vi "motor.vi"() -> ()   [LabVIEW 2018]
panel:
  out "返回值":string
  out "连接串口":string
  out "移动位置":string
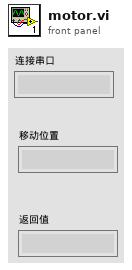
[diagram p1: front panel]
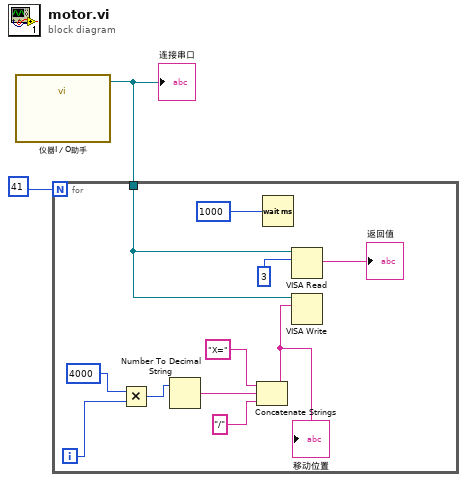
[diagram p0: block diagram]
diagram:
  n1 = call "仪器I／O助手"() -> ("Session Out"=w1:refnum<visa-resource-name>)  [unwired: 26 in, 1 out]
  "连接串口" <- w1
  n2 = for {
    N: 41 -> [_]
    tunnel: w1 -> [w7]
    i -> [w13]
    n3 = Multiply(x=4000, y=w13) -> (x*y=w9:i32)
    n4 = Number To Decimal String(number=w9) -> (decimal integer string=w3:string)  [unwired: 1 in]
    n5 = Concatenate Strings("X=", w3, "/") -> (w8:string)
    "移动位置" <- w8
    n6 = Wait (ms)(milliseconds to wait=1000) -> ()  [unwired: 1 out]
    n7 = VISA Read(VISA resource name=w7, byte count=3) -> (read buffer=→"返回值":string)  [unwired: 1 in, 3 out]
    n8 = VISA Write(VISA resource name=w7, write buffer=w8) -> ()  [unwired: 1 in, 3 out]
  }
